vi "Edit-SM1000-conversion-settings.vi"(8 "error in (no error)":errorcluster, 11 "Reference in":T4) -> (0 "error out":errorcluster, 3 "Reference out":T4)   [LabVIEW 2013, in "MaterialCharacterization.lvlib" / "MC-SM1000.lvclass"]
uses:
  MC-SM1000.lvclass
  Object-reference.ctl
  TCP-settings.ctl
  DOTNET-settings.ctl
  Device-identification.ctl
  MC-SM1000.lvclass/MC-SM1000.ctl
panel:
  in  "DOTNET settings":T1={"Target IP"="128.178.146.163", "Target broadcast port"=11000, "Target communication port"=12200, "clientID"=-1, "Broadcast IP"="224.168.100.2", "Servercount"=-1, "Device IDs"=[{"Name"="EC1000", "IP"="128.178.146.163", "Mac address"="mac"}]}
  in  "TCP settings":T3={"Target IP"="128.178.146.163", "Target TCP port"=12500, "TCP read mode"=enum."CRLF", "TCP read buffer"=4096, "Read timeout"=5000}
  in  "Cancel":bool
  in  "Ok":bool
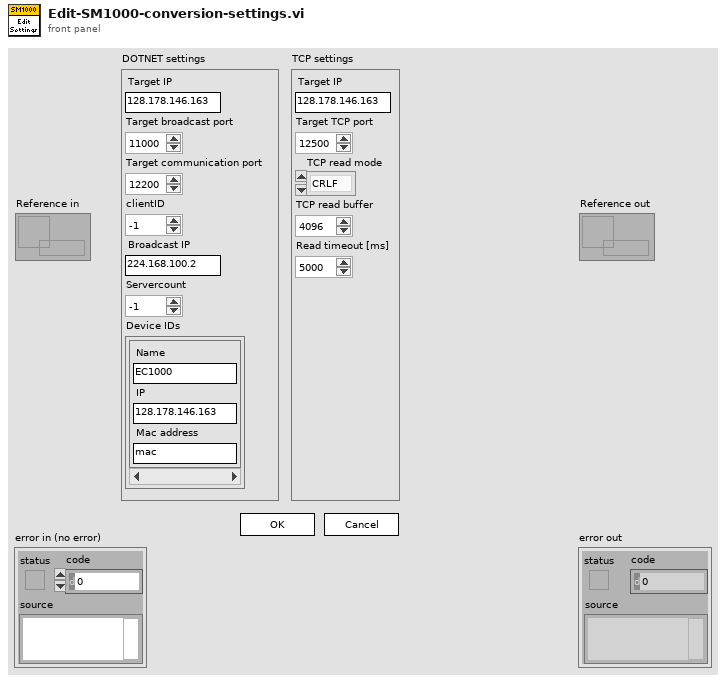
[diagram p1: front panel]
types:
  T1 = typedef "MaterialCharacterization.lvlib/MC-SM1000.lvclass/DOTNET-settings.ctl" = cluster{"Target IP":string, "Target broadcast port":i32, "Target communication port":i32, "clientID":i32, "Broadcast IP":string, "Servercount":i32, "Device IDs":T2[]}
  T2 = typedef "MaterialCharacterization.lvlib/MC-SM1000.lvclass/Device-identification.ctl" = cluster{"Name":string, "IP":string, "Mac address":string}
  T3 = typedef "MaterialCharacterization.lvlib/MC-SM1000.lvclass/TCP-settings.ctl" = cluster{"Target IP":string, "Target TCP port":u16, "TCP read mode":enum16{"Standard", "Buffered", "CRLF", "Immediate"}, "TCP read buffer":i32, "Read timeout":i32}
  T4 = typedef "MaterialCharacterization.lvlib/MC-SM1000.lvclass/Object-reference.ctl" = refnum<data-value>
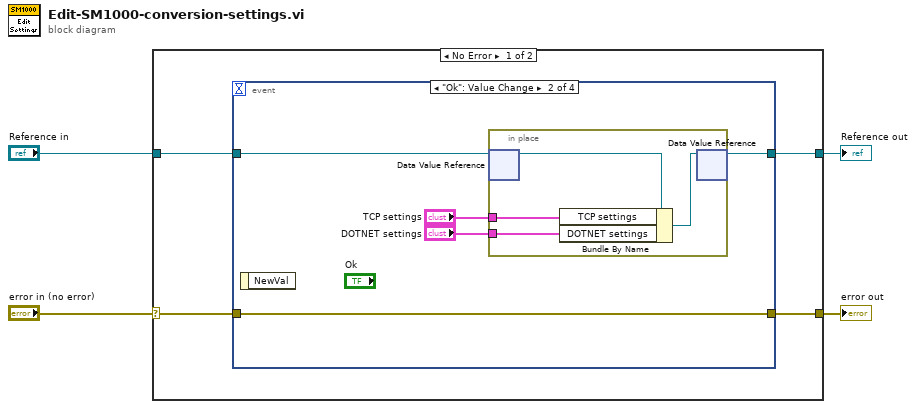
[diagram p0: block diagram]
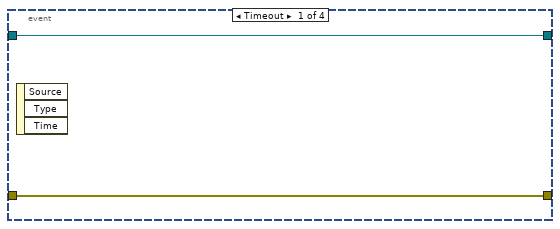
[diagram p2: hidden frame]
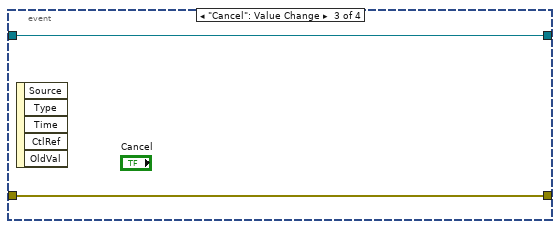
[diagram p3: hidden frame]
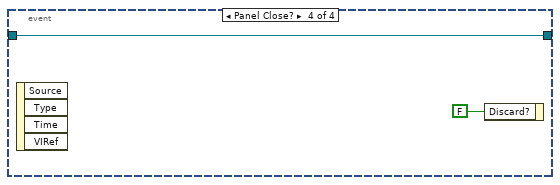
[diagram p4: hidden frame]
diagram:
  n1 = case shown="No Error" "error in (no error)" {
    selector: "error in (no error)" -> [w8 w24]
    tunnel: [w5 w24] -> w3
    tunnel: [w6 w25] -> w1
    tunnel: "Reference in" -> [w7 w25]
    frame No Error {
      n2 = event shown="[1] \"Ok\": Value Change" {
        selector: _ -> [_ _ _ _]
        dyn-events: _ -> [_ _ _ _]
        timeout: _ -> [_ _ _ _]
        tunnel: w8 -> [w10 w13 w21 _]
        tunnel: w7 -> [w9 w15 w20 w22]
        tunnel: [w9 w14 w20 w22] -> w6
        tunnel: [w10 w13 w21 _] -> w5
        event Timeout {
          n3 = event-data() -> ()  [unwired: 1 in, 3 out]
        }
        event "Ok": Value Change {
          n4 = event-data() -> ()  [unwired: 1 in, 1 out]
          n5 = in-place {
            in-place-border: "TCP settings" -> [w17]
            in-place-border: "DOTNET settings" -> [w16]
            n6 = in-place-dvr #1(w15) -> (w19:refnum<class "MC-SM1000.lvclass">)  [unwired: 1 out]
            n7 = Bundle By Name(cluster=w19, "TCP settings"=w17, "DOTNET settings"=w16) -> (w18:refnum<class "MC-SM1000.lvclass">)
            n8 = in-place-dvr #1(w18) -> (w14:T4)  [unwired: 1 out]
          }
        }
        event "Cancel": Value Change {
          n9 = event-data() -> ()  [unwired: 1 in, 5 out]
        }
        event Panel Close? {
          n10 = event-data() -> ()  [unwired: 1 in, 4 out]
          n11 = event-data("Discard?"=FALSE) -> ()  [unwired: 1 in, 1 out]
        }
      }
    }
    frame Error {
    }
  }
  "error out" <- w3
  "Reference out" <- w1
